vi "Construct Weather Forecast.vi"(5 "Weather Forecast In":refnum<class "Weather Forecast.lvclass">, 8 "error in (no error)":errorcluster, 11 "Date":timestamp) -> (0 "error out":errorcluster, 3 "Weather Forecast":refnum<class "Weather Forecast.lvclass">)   [LabVIEW 2017, in "Tests.lvlib" / "Weather Forecast.lvclass"]
uses:
  Weather Forecast.lvclass
  Weather Forecast.lvclass/Weather Forecast.ctl
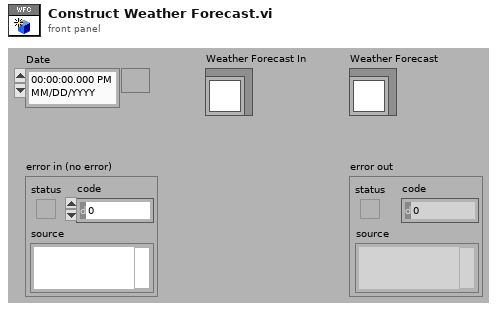
[diagram p1: front panel]
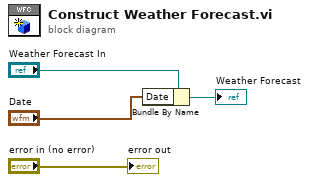
[diagram p0: block diagram]
diagram:
  n1 = Bundle By Name(cluster="Weather Forecast In", "Date"="Date") -> (→"Weather Forecast":refnum<class "Weather Forecast.lvclass">)
  "error out" <- "error in (no error)"
